vi "Scan.vi"() -> (0 "IR_D_Center":dbl)   [LabVIEW 2014]
panel:
  out "Waveform Chart":dynamicdata(graph)
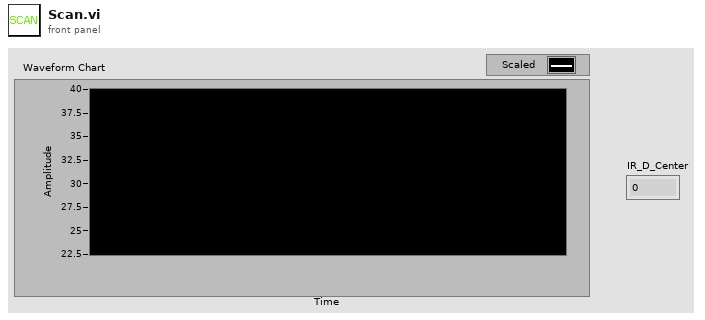
[diagram p1: front panel]
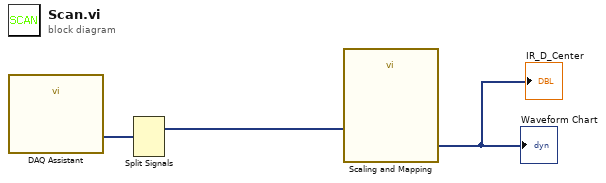
[diagram p0: block diagram]
diagram:
  n1 = call "DAQ Assistant"() -> ("data"=w3:dynamicdata)  [unwired: 17 in, 2 out]
  n2 = Split Signals(w3) -> (w1:dynamicdata)  [unwired: 5 in, 4 out]
  n3 = call "Scaling and Mapping"("Signals"=w1) -> ("Scaled Signals"=→"Waveform Chart" →"IR_D_Center":dynamicdata)  [unwired: 9 in, 1 out]
